vi "Add Tasks.vi"(8 "error in (no error)":errorcluster, 10 "User Selections":string[](array[string]), 11 "BuildServer in":refnum<class "BuildServer.lvclass">) -> (0 "error out":errorcluster, 3 "BuildServer out":refnum<class "BuildServer.lvclass">)   [LabVIEW 2017, in "BuildServer.lvlib" / "BuildServer.lvclass"]
uses:
  BuildServer.lvclass
  <vilib>/ActorFramework/Actor/Actor.lvclass
  BuildServer Messages/Update TaskView Msg/Update TaskView Msg.lvclass
  Volumes/Data/Users/benji667/Git/BuildFarm/WebSocket Server/Actors/Actor wHelper/Actor wHelper/Actor wHelper.lvclass
  Volumes/Data/Users/benji667/Git/BuildFarm/WebSocket Server/Actors/Actor wHelper/Actor wLauncher/Actor wLauncher.lvclass
  Volumes/Data/Users/benji667/Git/BuildFarm/WebSocket Server/Actors/Actor wHelper/Actor wUI/Actor wUI.lvclass
  Applications/National Instruments/LabVIEW 2017 64-bit/vi.lib/ActorFramework/Actor/Actor.lvclass
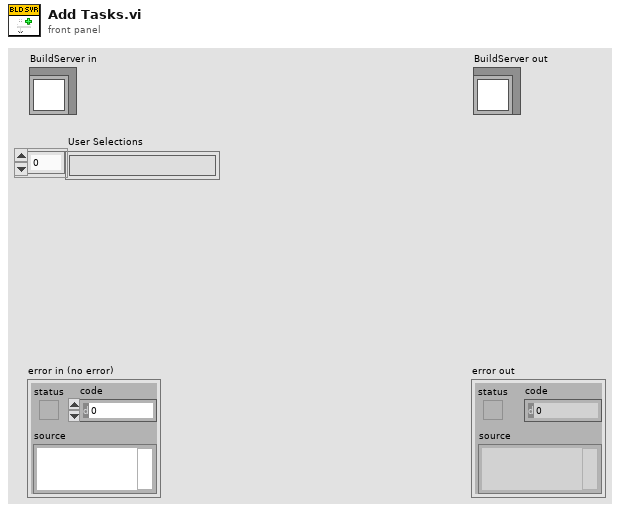
[diagram p1: front panel]
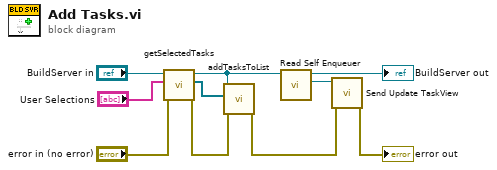
[diagram p0: block diagram]
diagram:
  n1 = call "getSelectedTasks.vi"("error in (no error)"="error in (no error)", "User Selections"="User Selections", "BuildServer in"="BuildServer in") -> ("error out"=w5:errorcluster, "Selected Tasks"=w6:refnum<class "Task.lvclass">[], "BuildServer out"=w4:refnum<class "BuildServer.lvclass">)  [unwired: 6 in]
  "BuildServer out" <- w4
  n2 = call "addTasksToList.vi"("error in (no error)"=w5, "Selected Tasks"=w6, "BuildServer in"=w4) -> ("error out"=w2:errorcluster)  [unwired: 8 in]
  n3 = call <vilib>:"Read Self Enqueuer.vi"("Actor"=w4) -> ("Self Enqueuer"=w3:refnum<class "Message Enqueuer.lvclass">)  [unwired: 10 in]
  n4 = call "Send Update TaskView.vi"("error in (no error)"=w2, "Message Enqueuer"=w3) -> ("error out"=→"error out":errorcluster)  [unwired: 8 in, 1 out]
